vi "TreeItem.Property.Get.vi"(8 "error in (no error)":errorcluster, 9 "Default Value":variant, 10 "Property Name":string, 11 "Basenode":refnum<k24>) -> (0 "error out":errorcluster, 1 "Variant":variant, 2 "Found?":bool, 3 "Basenode":refnum<k24>)   [LabVIEW 2015, in "Advanced System Definition.lvlib"]
uses:
  SysDef API/Advanced System Definition.lvlib
  NationalInstruments.VeriStand.SystemStorage
  _Types/Property.DependentFile.ctl
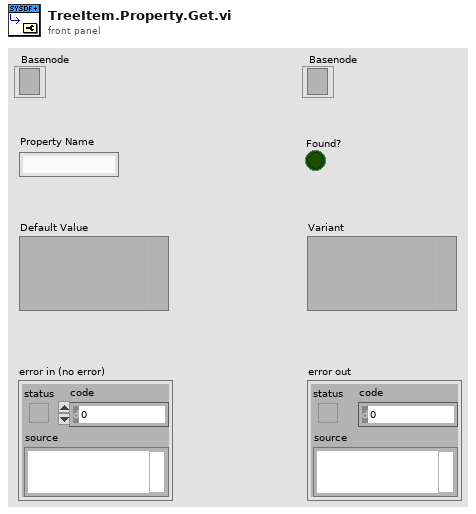
[diagram p1: front panel]
types:
  T1 = typedef "Advanced System Definition.lvlib/Property.DependentFile.ctl" = cluster{"Original Path":path, "Version":string, "RTDestination":path, "ForceDownload":bool, "SupportedTarget":string, "MD5":string}
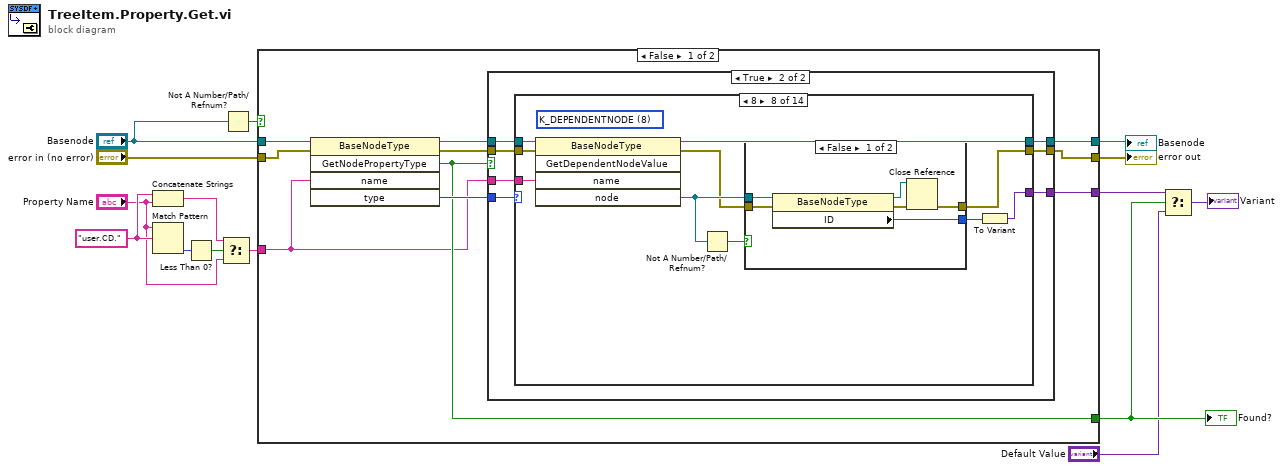
[diagram p0: block diagram]
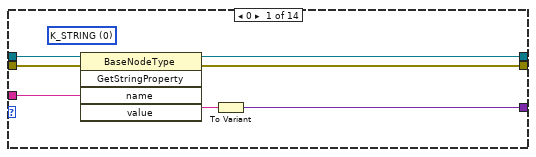
[diagram p3: hidden frame]
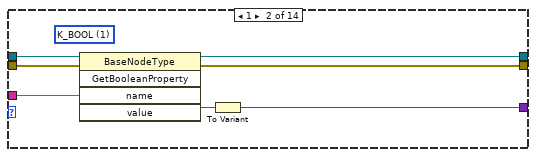
[diagram p4: hidden frame]
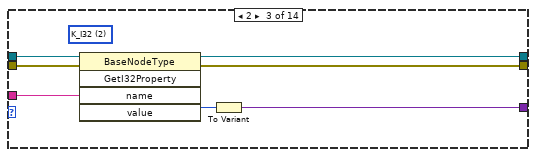
[diagram p5: hidden frame]
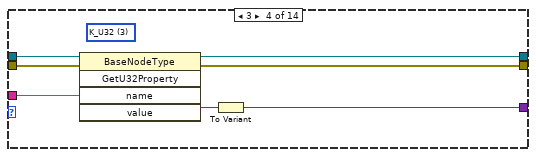
[diagram p6: hidden frame]
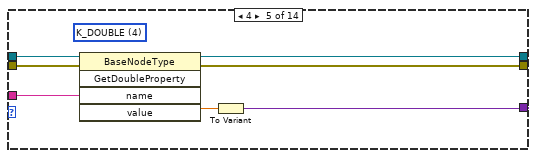
[diagram p7: hidden frame]
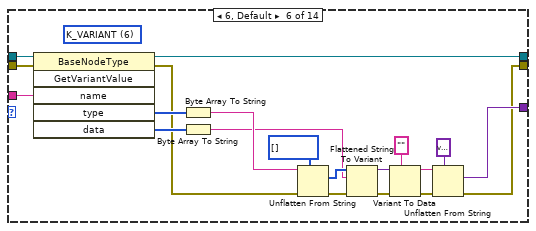
[diagram p8: hidden frame]
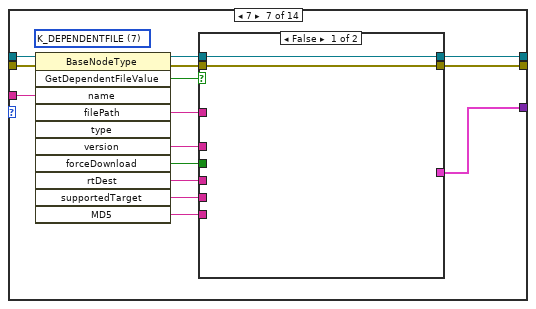
[diagram p9: hidden frame]
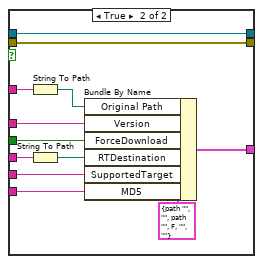
[diagram p10: hidden frame]
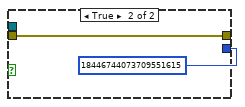
[diagram p11: hidden frame]
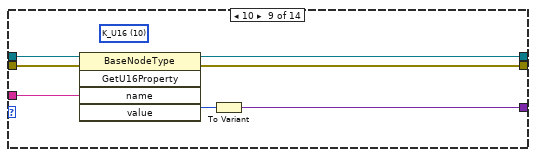
[diagram p12: hidden frame]
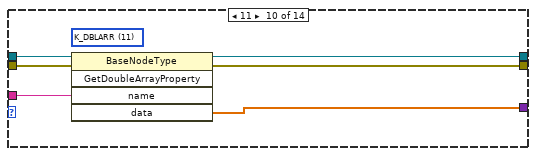
[diagram p13: hidden frame]
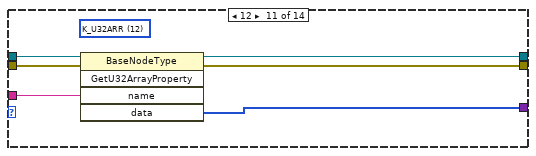
[diagram p14: hidden frame]
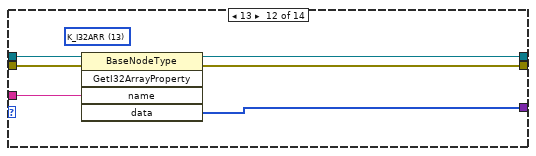
[diagram p15: hidden frame]
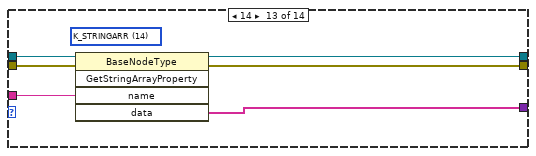
[diagram p16: hidden frame]
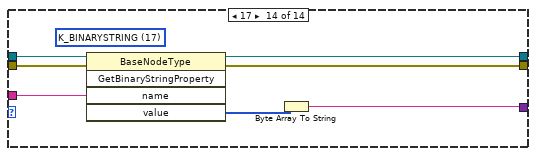
[diagram p17: hidden frame]
diagram:
  w3 = "user.CD." ("regular expression")
  n1 = Concatenate Strings(w3, "Property Name") -> (w4:string)
  n2 = Match Pattern(string="Property Name", regular expression=w3) -> (offset past match=w6:i32)  [unwired: 1 in, 3 out]
  n3 = Less Than 0?(x=w6) -> (x < 0?=w5:bool)
  n4 = Select(t=w4, s=w5, f="Property Name") -> (s? t:f=w1:string)
  n5 = Not A Number/Path/Refnum?(number/path/refnum="Basenode") -> (NaN/Path/Refnum?=w15:bool)
  n6 = case shown="False" w15 {
    tunnel: w1 -> [w16 _]
    tunnel: "Basenode" -> [w25 w176]
    tunnel: "error in (no error)" -> [w24 w175]
    tunnel: [w20 _] -> w12
    tunnel: [w19 _] -> w11
    tunnel: [w18 w176] -> w8
    tunnel: [w17 w175] -> w7
    frame False {
      n7 = invoke class="BaseNodeType" method="GetNodePropertyType"(reference=w25, error in=w24, "name"=w16) -> (reference out=w21:refnum<k24>, error out=w23:errorcluster, "GetNodePropertyType"=w20:bool, "type"=w22:i32)  [unwired: 2 in, 1 out]
      n8 = case shown="True" w20 {
        tunnel: [w26 w34] -> w18
        tunnel: [w27 w33] -> w17
        tunnel: [_ w32] -> w19
        tunnel: w23 -> [w27 w31]
        tunnel: w22 -> [_ w30]
        tunnel: w21 -> [w26 w29]
        tunnel: w16 -> [_ w28]
        frame False {
        }
        frame True {
          n9 = case shown="8" w30 {
            tunnel: [w41 w48 w55 w62 w69 w89 w91 w125 w143 w149 w155 w161 w163 w168] -> w34
            tunnel: w31 -> [w40 w47 w54 w61 w68 w88 w100 w128 w142 w148 w154 w160 w167 w173]
            tunnel: [w39 w46 w53 w60 w67 w71 w92 w120 w141 w147 w153 w159 w166 w169] -> w33
            tunnel: [w37 w44 w51 w58 w65 w72 w90 w124 w139 w146 w152 w158 w165 w170] -> w32
            tunnel: w29 -> [w35 w43 w49 w56 w63 w87 w101 w127 w138 w144 w151 w157 w162 w174]
            tunnel: w28 -> [w36 w42 w50 w57 w64 w86 w99 w126 w137 w145 w150 w156 w164 w172]
            frame 0 {
              (unwired) 0 items=["K_STRING", "K_BOOL", "K_I32", "K_U32", "K_DOUBLE", "K_U64", "K_VARIANT", "K_DEPENDENTFILE", "K_DEPENDENTNODE", "K_DATASOURCENODE", "K_U16", "K_DBLARR", "K_U32ARR", "K_I32ARR", "K_STRINGARR", "K_DICTIONARY", "K_DICTIONARYARR"] ("type")
              n10 = invoke class="BaseNodeType" method="GetStringProperty"(reference=w35, error in=w40, "name"=w36) -> (reference out=w41:refnum<k24>, error out=w39:errorcluster, "value"=w38:string)  [unwired: 2 in, 2 out]
              n11 = To Variant(anything=w38) -> (Variant=w37:variant)
            }
            frame 1 {
              (unwired) 1 items=["K_STRING", "K_BOOL", "K_I32", "K_U32", "K_DOUBLE", "K_U64", "K_VARIANT", "K_DEPENDENTFILE", "K_DEPENDENTNODE", "K_DATASOURCENODE", "K_U16", "K_DBLARR", "K_U32ARR", "K_I32ARR", "K_STRINGARR", "K_DICTIONARY", "K_DICTIONARYARR"] ("type")
              n12 = invoke class="BaseNodeType" method="GetBooleanProperty"(reference=w43, error in=w47, "name"=w42) -> (reference out=w48:refnum<k24>, error out=w46:errorcluster, "value"=w45:bool)  [unwired: 2 in, 2 out]
              n13 = To Variant(anything=w45) -> (Variant=w44:variant)
            }
            frame 2 {
              (unwired) 2 items=["K_STRING", "K_BOOL", "K_I32", "K_U32", "K_DOUBLE", "K_U64", "K_VARIANT", "K_DEPENDENTFILE", "K_DEPENDENTNODE", "K_DATASOURCENODE", "K_U16", "K_DBLARR", "K_U32ARR", "K_I32ARR", "K_STRINGARR", "K_DICTIONARY", "K_DICTIONARYARR"] ("type")
              n14 = invoke class="BaseNodeType" method="GetI32Property"(reference=w49, error in=w54, "name"=w50) -> (reference out=w55:refnum<k24>, error out=w53:errorcluster, "value"=w52:i32)  [unwired: 2 in, 2 out]
              n15 = To Variant(anything=w52) -> (Variant=w51:variant)
            }
            frame 3 {
              (unwired) 3 items=["K_STRING", "K_BOOL", "K_I32", "K_U32", "K_DOUBLE", "K_U64", "K_VARIANT", "K_DEPENDENTFILE", "K_DEPENDENTNODE", "K_DATASOURCENODE", "K_U16", "K_DBLARR", "K_U32ARR", "K_I32ARR", "K_STRINGARR", "K_DICTIONARY", "K_DICTIONARYARR"] ("type")
              n16 = invoke class="BaseNodeType" method="GetU32Property"(reference=w56, error in=w61, "name"=w57) -> (reference out=w62:refnum<k24>, error out=w60:errorcluster, "value"=w59:u32)  [unwired: 2 in, 2 out]
              n17 = To Variant(anything=w59) -> (Variant=w58:variant)
            }
            frame 4 {
              (unwired) 4 items=["K_STRING", "K_BOOL", "K_I32", "K_U32", "K_DOUBLE", "K_U64", "K_VARIANT", "K_DEPENDENTFILE", "K_DEPENDENTNODE", "K_DATASOURCENODE", "K_U16", "K_DBLARR", "K_U32ARR", "K_I32ARR", "K_STRINGARR", "K_DICTIONARY", "K_DICTIONARYARR"] ("type")
              n18 = invoke class="BaseNodeType" method="GetDoubleProperty"(reference=w63, error in=w68, "name"=w64) -> (reference out=w69:refnum<k24>, error out=w67:errorcluster, "value"=w66:dbl)  [unwired: 2 in, 2 out]
              n19 = To Variant(anything=w66) -> (Variant=w65:variant)
            }
            frame 6, Default {
              (unwired) 6 items=["K_STRING", "K_BOOL", "K_I32", "K_U32", "K_DOUBLE", "K_U64", "K_VARIANT", "K_DEPENDENTFILE", "K_DEPENDENTNODE", "K_DATASOURCENODE", "K_U16", "K_DBLARR", "K_U32ARR", "K_I32ARR", "K_STRINGARR", "K_DICTIONARY", "K_DICTIONARYARR"] ("type")
              n20 = invoke class="BaseNodeType" method="GetVariantValue"(reference=w87, error in=w88, "name"=w86) -> (reference out=w89:refnum<k24>, error out=w70:errorcluster, "type"=w73:u8[], "data"=w74:u8[])  [unwired: 3 in, 2 out]
              n21 = Byte Array To String(unsigned byte array=w73) -> (string=w82:string)
              n22 = Byte Array To String(unsigned byte array=w74) -> (string=w81:string)
              n23 = Unflatten From String(type=i16[] [] ("type string"), binary string=w82, error in (no error)=w70) -> (value=w84:i16[], error out=w83:errorcluster)  [unwired: 2 in, 1 out]
              n24 = Flattened String To Variant(4:w83, 6:w81, 7:w84) -> (0:w77:errorcluster, 3:w80:variant)
              n25 = Variant To Data(error in=w77, type="", Variant=w80) -> (data=w78:string, error out=w76:errorcluster)
              n26 = Unflatten From String(type=variant ("variant"), binary string=w78, error in (no error)=w76) -> (value=w72:variant, error out=w71:errorcluster)  [unwired: 2 in, 1 out]
            }
            frame 7 {
              (unwired) 7 items=["K_STRING", "K_BOOL", "K_I32", "K_U32", "K_DOUBLE", "K_U64", "K_VARIANT", "K_DEPENDENTFILE", "K_DEPENDENTNODE", "K_DATASOURCENODE", "K_U16", "K_DBLARR", "K_U32ARR", "K_I32ARR", "K_STRINGARR", "K_DICTIONARY", "K_DICTIONARYARR"] ("type")
              n27 = invoke class="BaseNodeType" method="GetDependentFileValue"(reference=w101, error in=w100, "name"=w99) -> (reference out=w103:refnum<k24>, error out=w102:errorcluster, "GetDependentFileValue"=w104:bool, "filePath"=w98:string, "version"=w97:string, "forceDownload"=w95:bool, "rtDest"=w96:string, "supportedTarget"=w94:string, "MD5"=w93:string)  [unwired: 8 in, 2 out]
              n28 = case shown="False" w104 {
                tunnel: [w105 w109] -> w92
                tunnel: [w106 w115] -> w91
                tunnel: [_ w118] -> w90
                tunnel: w102 -> [w105 w109]
                tunnel: w103 -> [w106 w115]
                tunnel: w98 -> [_ w114]
                tunnel: w97 -> [_ w113]
                tunnel: w96 -> [_ w112]
                tunnel: w95 -> [_ w108]
                tunnel: w94 -> [_ w111]
                tunnel: w93 -> [_ w110]
                frame False {
                }
                frame True {
                  n29 = String To Path(string=w114) -> (path=w107:path)
                  n30 = String To Path(string=w112) -> (path=w116:path)
                  n31 = Bundle By Name(cluster=T1 {"Original Path"=path "", "Version"="", "RTDestination"=path "", "ForceDownload"=FALSE, "SupportedTarget"="", "MD5"=""} ("OptionalInfo"), "Original Path"=w107, "Version"=w113, "ForceDownload"=w108, "RTDestination"=w116, "SupportedTarget"=w111, "MD5"=w110) -> (w118:T1)
                }
              }
            }
            frame 8 {
              (unwired) 8 items=["K_STRING", "K_BOOL", "K_I32", "K_U32", "K_DOUBLE", "K_U64", "K_VARIANT", "K_DEPENDENTFILE", "K_DEPENDENTNODE", "K_DATASOURCENODE", "K_U16", "K_DBLARR", "K_U32ARR", "K_I32ARR", "K_STRINGARR", "K_DICTIONARY", "K_DICTIONARYARR"] ("type")
              n32 = invoke class="BaseNodeType" method="GetDependentNodeValue"(reference=w127, error in=w128, "name"=w126) -> (reference out=w125:refnum<k24>, error out=w121:errorcluster, "node"=w122:refnum<k24>)  [unwired: 2 in, 2 out]
              n33 = Not A Number/Path/Refnum?(number/path/refnum=w122) -> (NaN/Path/Refnum?=w123:bool)
              n34 = case shown="False" w123 {
                tunnel: w121 -> [w129 w136]
                tunnel: [w130 w136] -> w120
                tunnel: w122 -> [w131 _]
                tunnel: [w134 u64 18446744073709551615 ("NodePtr")] -> w119
                frame False {
                  n35 = property class="BaseNodeType"(reference=w131, error in=w129) -> (reference out=w132:refnum<k24>, error out=w133:errorcluster, "ID"=w134:u64)
                  n36 = Close Reference(reference=w132, error in (no error)=w133) -> (error out=w130:errorcluster)
                }
                frame True {
                }
              }
              n37 = To Variant(anything=w119) -> (Variant=w124:variant)
            }
            frame 10 {
              (unwired) 10 items=["K_STRING", "K_BOOL", "K_I32", "K_U32", "K_DOUBLE", "K_U64", "K_VARIANT", "K_DEPENDENTFILE", "K_DEPENDENTNODE", "K_DATASOURCENODE", "K_U16", "K_DBLARR", "K_U32ARR", "K_I32ARR", "K_STRINGARR", "K_DICTIONARY", "K_DICTIONARYARR"] ("type")
              n38 = invoke class="BaseNodeType" method="GetU16Property"(reference=w138, error in=w142, "name"=w137) -> (reference out=w143:refnum<k24>, error out=w141:errorcluster, "value"=w140:u16)  [unwired: 2 in, 2 out]
              n39 = To Variant(anything=w140) -> (Variant=w139:variant)
            }
            frame 11 {
              (unwired) 11 items=["K_STRING", "K_BOOL", "K_I32", "K_U32", "K_DOUBLE", "K_U64", "K_VARIANT", "K_DEPENDENTFILE", "K_DEPENDENTNODE", "K_DATASOURCENODE", "K_U16", "K_DBLARR", "K_U32ARR", "K_I32ARR", "K_STRINGARR", "K_DICTIONARY", "K_DICTIONARYARR"] ("type")
              n40 = invoke class="BaseNodeType" method="GetDoubleArrayProperty"(reference=w144, error in=w148, "name"=w145) -> (reference out=w149:refnum<k24>, error out=w147:errorcluster, "data"=w146:dbl[])  [unwired: 2 in, 2 out]
            }
            frame 12 {
              (unwired) 12 items=["K_STRING", "K_BOOL", "K_I32", "K_U32", "K_DOUBLE", "K_U64", "K_VARIANT", "K_DEPENDENTFILE", "K_DEPENDENTNODE", "K_DATASOURCENODE", "K_U16", "K_DBLARR", "K_U32ARR", "K_I32ARR", "K_STRINGARR", "K_DICTIONARY", "K_DICTIONARYARR"] ("type")
              n41 = invoke class="BaseNodeType" method="GetU32ArrayProperty"(reference=w151, error in=w154, "name"=w150) -> (reference out=w155:refnum<k24>, error out=w153:errorcluster, "data"=w152:u32[])  [unwired: 2 in, 2 out]
            }
            frame 13 {
              (unwired) 13 items=["K_STRING", "K_BOOL", "K_I32", "K_U32", "K_DOUBLE", "K_U64", "K_VARIANT", "K_DEPENDENTFILE", "K_DEPENDENTNODE", "K_DATASOURCENODE", "K_U16", "K_DBLARR", "K_U32ARR", "K_I32ARR", "K_STRINGARR", "K_DICTIONARY", "K_DICTIONARYARR"] ("type")
              n42 = invoke class="BaseNodeType" method="GetI32ArrayProperty"(reference=w157, error in=w160, "name"=w156) -> (reference out=w161:refnum<k24>, error out=w159:errorcluster, "data"=w158:i32[])  [unwired: 2 in, 2 out]
            }
            frame 14 {
              (unwired) 14 items=["K_STRING", "K_BOOL", "K_I32", "K_U32", "K_DOUBLE", "K_U64", "K_VARIANT", "K_DEPENDENTFILE", "K_DEPENDENTNODE", "K_DATASOURCENODE", "K_U16", "K_DBLARR", "K_U32ARR", "K_I32ARR", "K_STRINGARR", "K_DICTIONARY", "K_DICTIONARYARR"] ("type")
              n43 = invoke class="BaseNodeType" method="GetStringArrayProperty"(reference=w162, error in=w167, "name"=w164) -> (reference out=w163:refnum<k24>, error out=w166:errorcluster, "data"=w165:string[])  [unwired: 2 in, 2 out]
            }
            frame 17 {
              (unwired) 17 items=["K_STRING", "K_BOOL", "K_I32", "K_U32", "K_DOUBLE", "K_U64", "K_VARIANT", "K_DEPENDENTFILE", "K_DEPENDENTNODE", "K_DATASOURCENODE", "K_U16", "K_DBLARR", "K_U32ARR", "K_I32ARR", "K_STRINGARR", "K_DICTIONARY", "K_DICTIONARYARR", "K_BINARYSTRING"] ("type")
              n44 = invoke class="BaseNodeType" method="GetBinaryStringProperty"(reference=w174, error in=w173, "name"=w172) -> (reference out=w168:refnum<k24>, error out=w169:errorcluster, "value"=w171:u8[])  [unwired: 2 in, 2 out]
              n45 = Byte Array To String(unsigned byte array=w171) -> (string=w170:string)
            }
          }
        }
      }
    }
    frame True {
    }
  }
  "Basenode" <- w8
  "Found?" <- w12
  "error out" <- w7
  n46 = Select(t=w11, s=w12, f="Default Value") -> (s? t:f=→"Variant":variant)
